vi "MCL Current Min Max Theta Y.vi"(8 "error in (no error)":errorcluster, 9 "handle":i32, 10 "max":dbl, 11 "min":dbl) -> (0 "error out":errorcluster, 1 "function return":i32, 2 "max out":dbl, 3 "min out":dbl)   [LabVIEW 2014, in "Madlib.lvlib"]
doc: "MADLIB_API int MCL_CurrentMinMaxThetaY(double *min, double *max, int handle);"
uses:
  <userlib>/Lambda2/lib/Madlib/Madlib.lvlib
  <userlib>/Lambda2/lib/Madlib/Madlib.dll
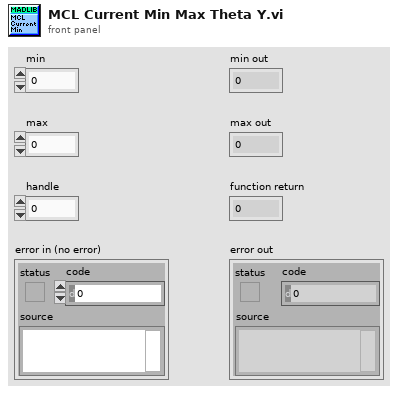
[diagram p1: front panel]
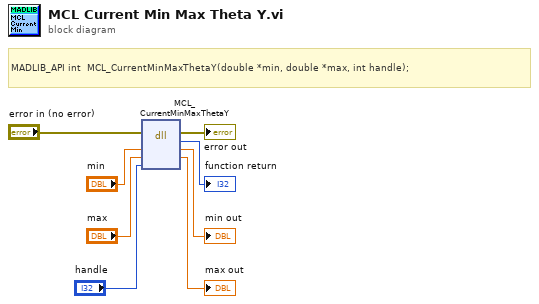
[diagram p0: block diagram]
diagram:
  # "MADLIB_API\tint\t\tMCL_CurrentMinMaxThetaY(double *min, double *max, int handle);"
  n1 = dll-call lib="C:/Program Files (x86)/National Instruments/LabVIEW 2014/user.lib/Lambda2/lib/Madlib/Madlib.*" fn="MCL_CurrentMinMaxThetaY"(error in="error in (no error)", "min"="min", "max"="max", "handle"="handle") -> (error out=→"error out":errorcluster, →"function return":i32, "min"=→"min out":dbl, "max"=→"max out":dbl)  [unwired: 3 in, 1 out]
